vi "Needle_controller_tester.vi"() -> ()   [LabVIEW 2018]
uses:
  <vilib>/Analysis/baseanly.llb/A x Vector.vi
  <vilib>/Analysis/NI_AALBase.lvlib
panel:
  in  "Rate":u8(ring)=15 items=["ADC18_DATA_RATE_1_SPS", "ADC18_DATA_RATE_3_SPS", "ADC18_DATA_RATE_5_SPS", "ADC18_DATA_RATE_10_SPS", "ADC18_DATA_RATE_13_SPS", "ADC18_DATA_RATE_15_SPS", "ADC18_DATA_RATE_50_SPS", "ADC18_DATA_RATE_60_SPS", "ADC18_DATA_RATE_150_SPS", "ADC18_DATA_RATE_300_SPS", "ADC18_DATA_RATE_900_SPS", "ADC18_DATA_RATE_1800_SPS", "ADC18_DATA_RATE_2880_SPS", "ADC18_DATA_RATE_5760_SPS", "ADC18_DATA_RATE_11520_SPS", "ADC18_DATA_RATE_23040_SPS"]
  in  "Mode":u8(ring)=2 items=["CONTINUOUS", "CONTINUOUS 2", "SINGLE_CYCLE", "CONT_SINGLE_CYCLE"]
  in  "Set ADC Data Rate":bool
  in  "Samples To Average":u8=3
  in  "Get All Sensor Data Continuous":bool
  out "All Data 2":T1={"Time"=713, "FT Data"={"xForce"=0.14730099, "yForce"=0.008982421, "zForce"=0.2579272, "xTorque"=-0.9978087, "yTorque"=-0.58180696, "zTorque"=-0.619802}, "Encoder Data"={"xPos"=0.0, "yPos"=0.0, "zPos"=0.0}}
  out "Encoder Data":cluster{"xPos":sgl, "yPos":sgl, "zPos":sgl}
  in  "Get Encoder Sensor Data":bool
  out "All Data":T1={"Time"=992, "FT Data"={"xForce"=0.14789405, "yForce"=0.009089709, "zForce"=0.2569944, "xTorque"=-0.9979577, "yTorque"=-0.58224803, "zTorque"=-0.6196828}, "Encoder Data"={"xPos"=0.0, "yPos"=0.0, "zPos"=0.0}}
  in  "Get All Sensor Data":bool
  in  "Set ADC Conversion Mode":bool
  in  "Check ADC":bool
  in  "Reset ADC":bool
  out "Calibrated":dbl[](array[numeric]) format="%.2f"
  out "Sensor Data":T2
  out "System Status":cluster{"boardState":u8}
  in  "Get FT Sensor Data":bool
  out "Error Code":T3(ring)
  out "Return FID":u8=4
  out "FID":u8=5
  in  "IP Address":string="192.168.5.101"
  out "System Info":T4={"fwVersion"="1.0", "pumpId"="NeedleController01", "ipAddr"="192.168.5.101", "macAddr"="3e:43:d3:26:35:fe"}
  out "error out":errorcluster
  in  "Get System Info":bool
  in  "Get System Status":bool
  in  "Stop":bool
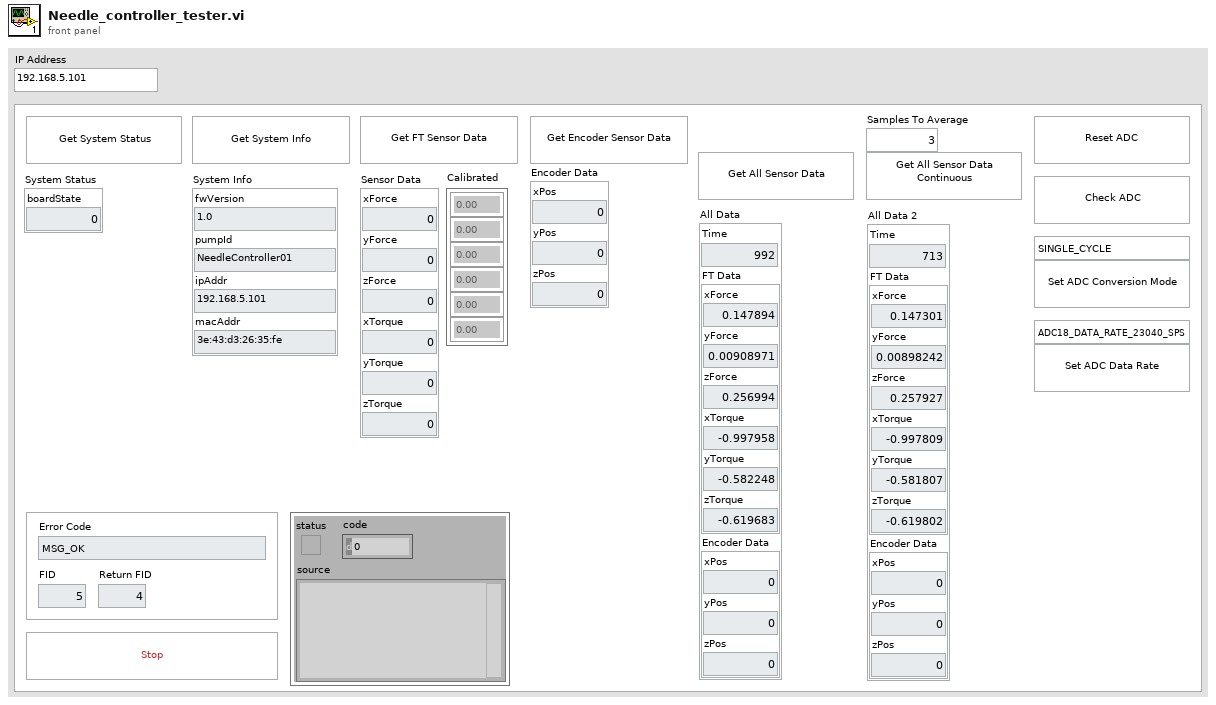
[diagram p1: front panel]
types:
  T1 = cluster{"Time":i32, "FT Data":cluster{"xForce":sgl, "yForce":sgl, "zForce":sgl, "xTorque":sgl, "yTorque":sgl, "zTorque":sgl}, "Encoder Data":cluster{"xPos":sgl, "yPos":sgl, "zPos":sgl}}
  T2 = cluster{"xForce":sgl, "yForce":sgl, "zForce":sgl, "xTorque":sgl, "yTorque":sgl, "zTorque":sgl}
  T3 = enum8{"MSG_OK", "MSG_ERROR_NOT_SUPPORTED", "MSG_ERROR_SENSOR_DISCONNECTED", "MSG_ERROR_READING_PENDING"}
  T4 = cluster{"fwVersion":string, "pumpId":string, "ipAddr":string, "macAddr":string}
  T5 = cluster{"fwVersion":string, "pumpId":string, "macAddr":string, "ipAddr":string}
  T6 = enum16{"big-endian, network order", "native, host order", "little-endian"}
  T7 = cluster{i32, "Sensor Data":cluster{"xForce":sgl, "yForce":sgl, "zForce":sgl, "xTorque":sgl, "yTorque":sgl, "zTorque":sgl}, "Sensor Data 2":cluster{"xForce":sgl, "yForce":sgl, "zForce":sgl}}
  T8 = cluster{"pumpState":i32, "suppliedVolume_ml":sgl, "flowRate_mlmin":sgl, "home":i32, "port":i32}
  T9 = cluster{"connection ID":refnum<k5>, "header length":u16}
  T10 = cluster{"boardState":u8, "tempSetpoint":sgl, "pH connected":bool, "Temp connected":bool, "pidOutput":dbl, "pidIntegral":dbl, "pidSetpoint":sgl, "pidStep":sgl, "pidMethod":u8}
  T11 = cluster{"header":cluster{"length":u16, "fid":u8, "error":u8}}
  T12 = cluster{"header":cluster{"length":u16, "fid":u8, "error":u8}, "Samples To Average":u8}
  T13 = cluster{"header":cluster{"length":u16, "fid":u8, "error":u8}, "Mode":u8}
  T14 = cluster{"header":cluster{"length":u16, "fid":u8, "error":u8}, "Rate":u8}
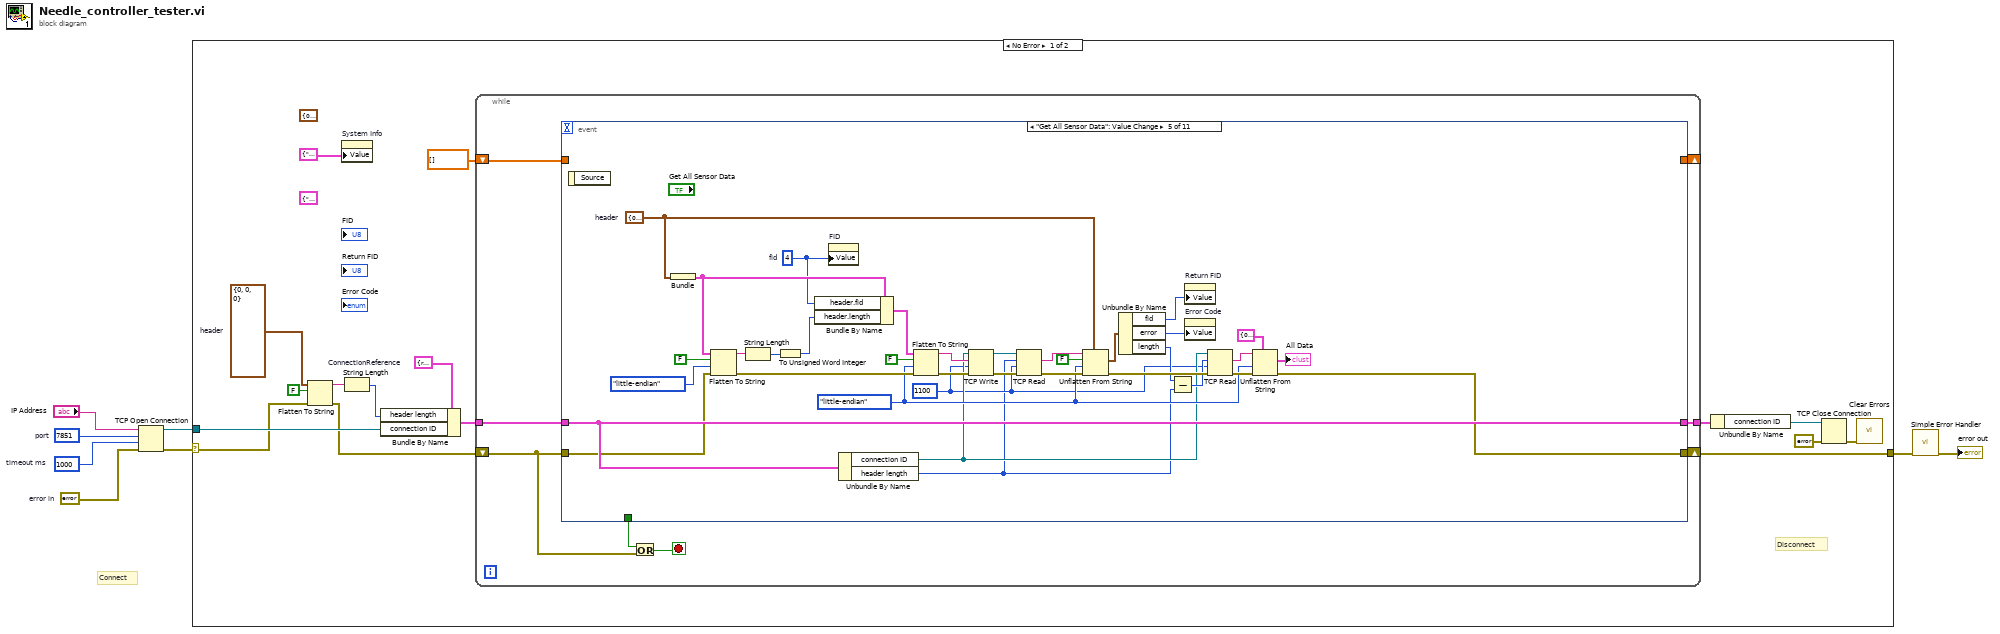
[diagram p0: block diagram]
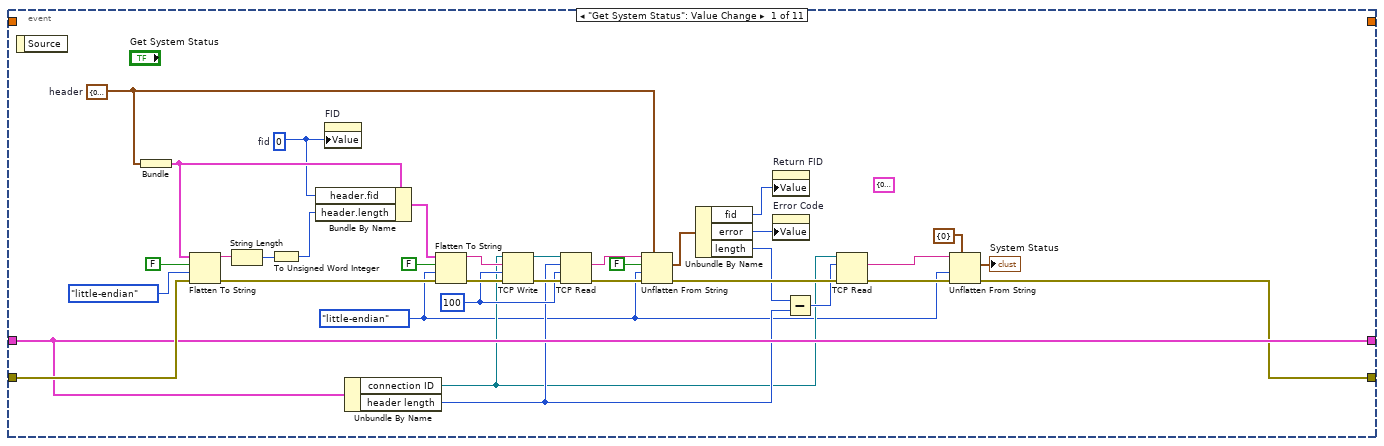
[diagram p2: hidden frame]
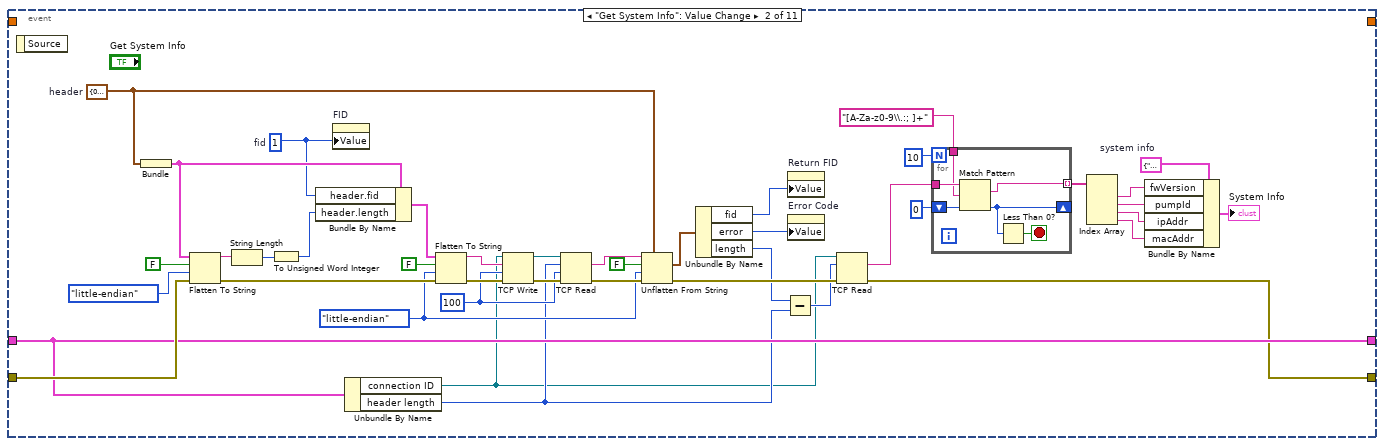
[diagram p3: hidden frame]
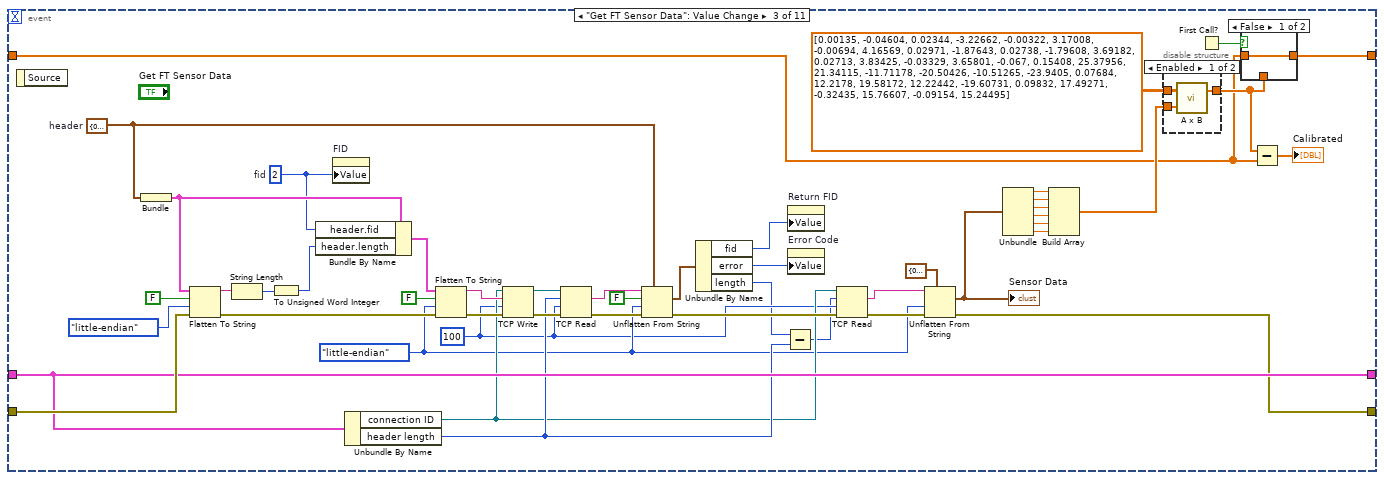
[diagram p4: hidden frame]
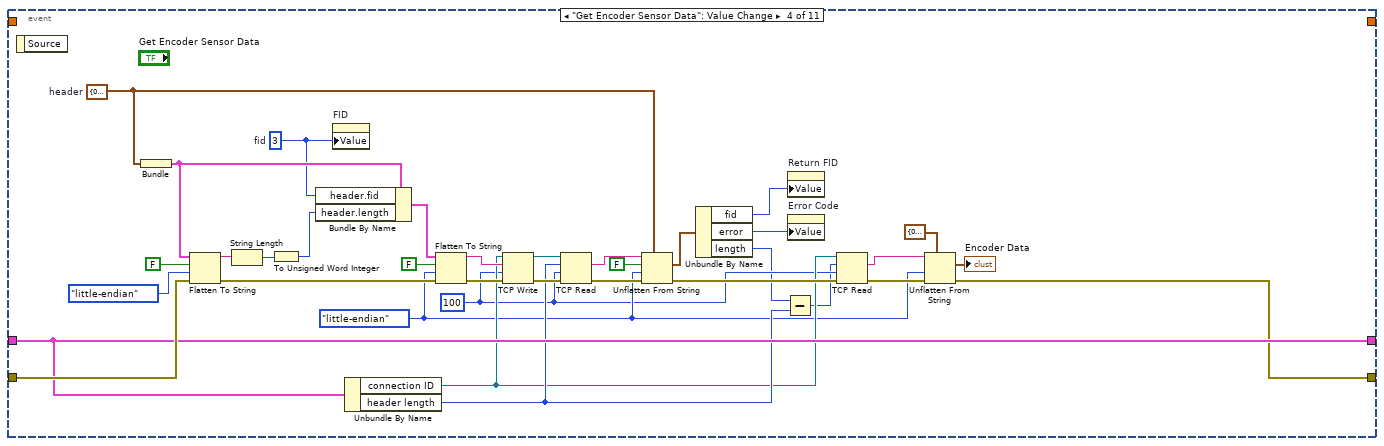
[diagram p7: hidden frame]
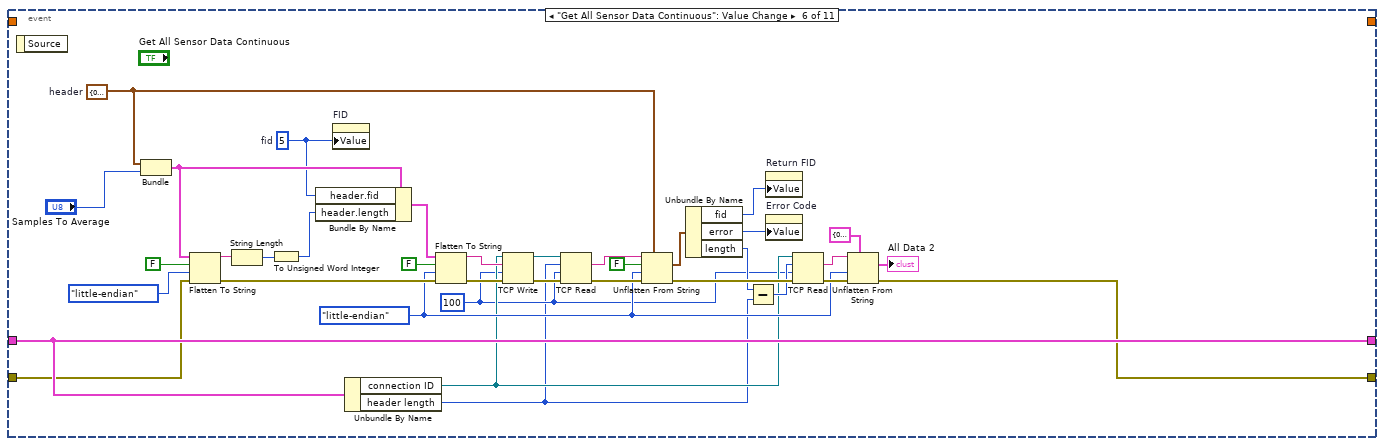
[diagram p8: hidden frame]
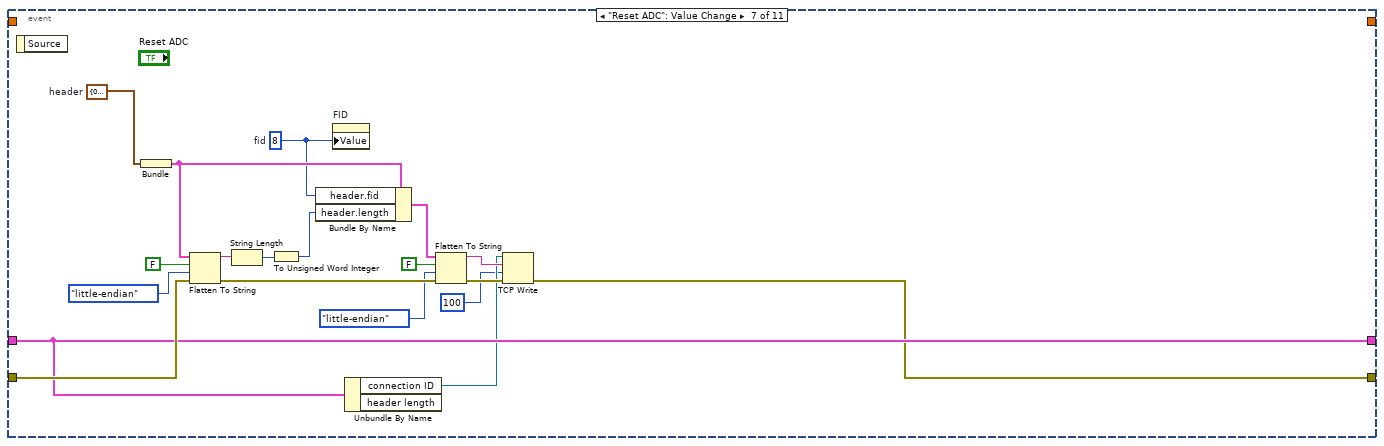
[diagram p9: hidden frame]
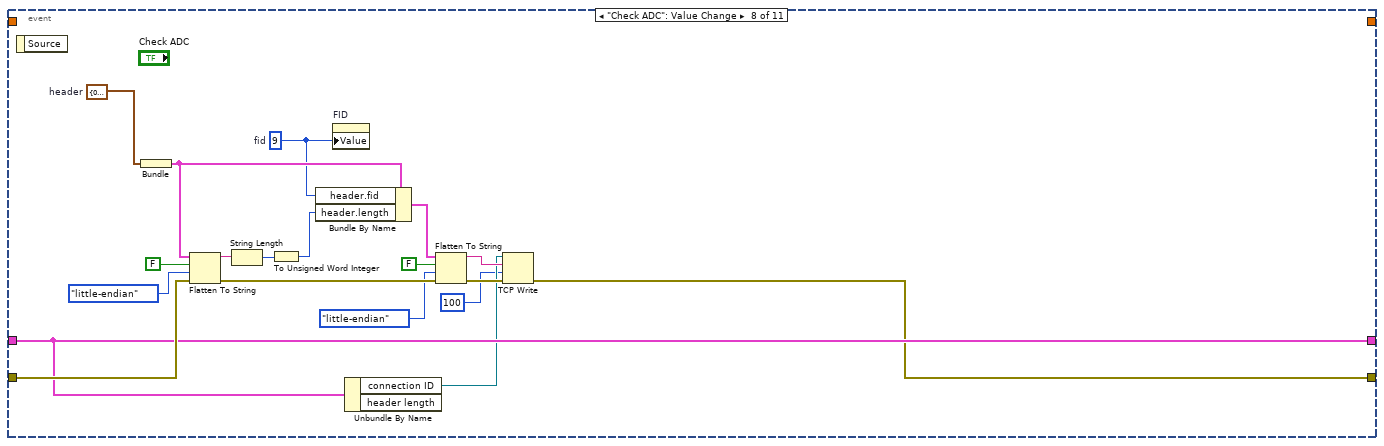
[diagram p10: hidden frame]
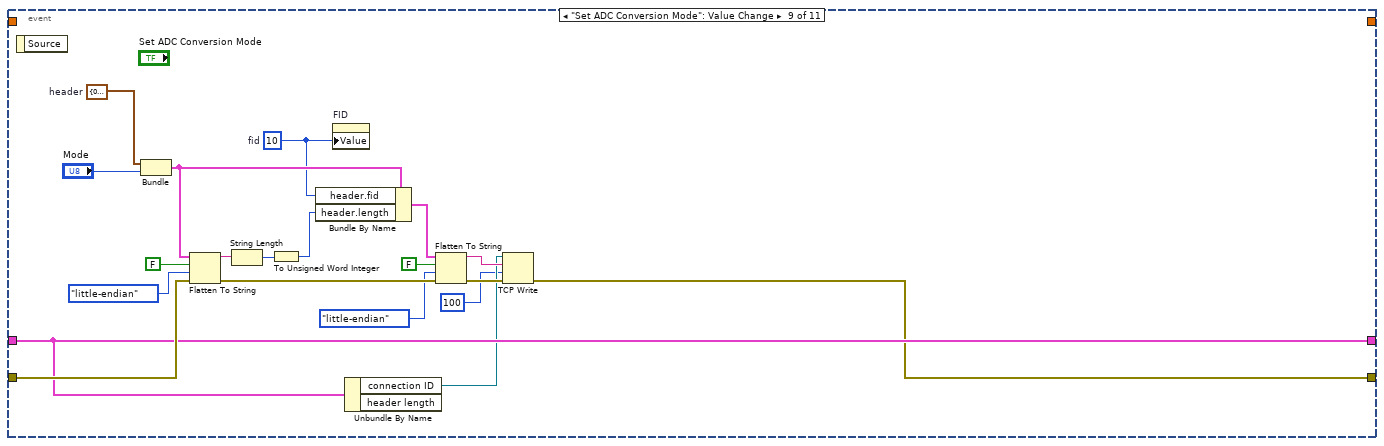
[diagram p11: hidden frame]
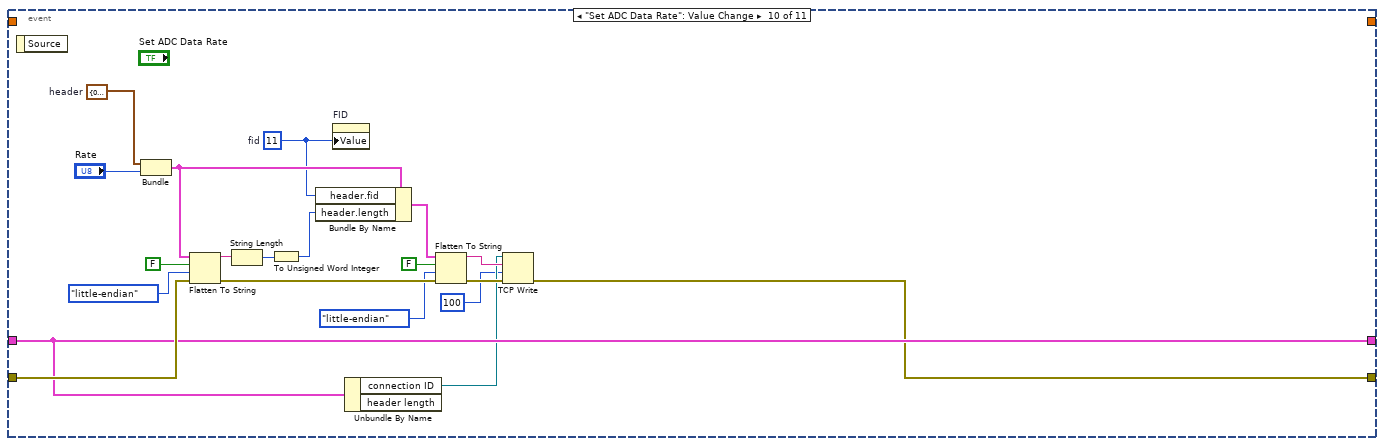
[diagram p12: hidden frame]
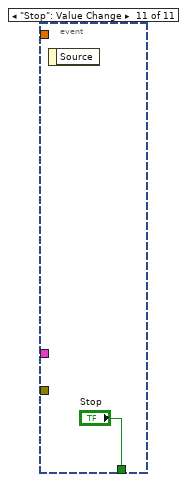
[diagram p13: hidden frame]
diagram:
  w6 = errorcluster {"status"=FALSE, "code"=0, "source"=""}  # error in
  w7 = 1000  # timeout ms
  w8 = u16 7851  # port
  # "Connect"
  n1 = TCP Open Connection(address="IP Address", remote port or service name=w8, timeout ms (60000)=w7, error in (no error)=w6) -> (connection ID=w5:refnum<k5>, error out=w1:errorcluster)  [unwired: 1 in]
  n2 = case shown="No Error" w1 {
    selector: w1 -> [w11 w355]
    tunnel: w5 -> [w20 _]
    tunnel: [w12 w355] -> w2
    frame No Error {
      (unwired) cluster{"axis":string, "stepPeriod (ms)":string} {"axis"="", "stepPeriod (ms)"=""} ("Return Motor Config")
      (unwired) T8 {"pumpState"=0, "suppliedVolume_ml"=0.0, "flowRate_mlmin"=0.0, "home"=0, "port"=0} ("Status")
      w19 = cluster{"length":u16, "fid":u8, "error":u8} {"length"=0, "fid"=0, "error"=0}  # header
      w21 = T9 {"connection ID"=refnum, "header length"=0}  # ConnectionReference
      # "Disconnect"
      n3 = Flatten To String(anything=w19, prepend array or string size? (T)=FALSE, error in (no error)=w11) -> (data string=w17:string, error out=w13:errorcluster)  [unwired: 1 in, 1 out]
      n4 = property on="System Info" class="Clust (strict)"("Value"=T5 {"fwVersion"="", "pumpId"="", "macAddr"="", "ipAddr"=""} ("system info")) -> ()  [unwired: 2 in, 2 out]
      n5 = String Length(string=w17) -> (length=w16:i32)
      n6 = Bundle By Name(cluster=w21, "header length"=w16, "connection ID"=w20) -> (w15:T9)
      n7 = while {
        tunnel: w15 -> [w32]
        tunnel: [w31] -> w14
        shift-right: [w30] -> w12
        shift-left: w13 -> [w28]
        shift-right: [w26] -> _
        shift-left: dbl[] [] ("A x Vector") -> [w25]
        stop <- w29 stop-if-true
        n8 = event shown="[4] \"Get All Sensor Data\": Value Change" {
          selector: _ -> [_ _ _ _ _ _ _ _ _ _ _]
          dyn-events: _ -> [_ _ _ _ _ _ _ _ _ _ _]
          timeout: _ -> [_ _ _ _ _ _ _ _ _ _ _]
          tunnel: w32 -> [w56 w98 w152 w193 w229 w265 w283 w302 w322 w342 _]
          tunnel: [w56 w98 w152 w193 w229 w265 w283 w302 w322 w342 _] -> w31
          tunnel: w28 -> [w57 w99 w153 w194 w206 w242 w284 w303 w323 w343 _]
          tunnel: [w39 w75 w136 w177 w207 w243 w276 w295 w315 w335 _] -> w30
          tunnel: [_ _ _ _ _ _ _ _ _ _ "Stop"] -> w27
          tunnel: [_ _ w119 _ _ _ _ _ _ _ _] -> w26
          tunnel: w25 -> [_ _ w117 _ _ _ _ _ _ _ _]
          event "Get System Status": Value Change {
            (unwired) T10 {"boardState"=0, "tempSetpoint"=0.0, "pH connected"=FALSE, "Temp connected"=FALSE, "pidOutput"=0.0, "pidIntegral"=0.0, "pidSetpoint"=0.0, "pidStep"=0.0, "pidMethod"=0} ("Status")
            w48 = cluster{"length":u16, "fid":u8, "error":u8} {"length"=0, "fid"=0, "error"=0}  # header
            w50 = 100 ("timeout ms (25000)")
            w36 = u8 0  # fid
            w38 = T6."little-endian" ("byte order (0:big-endian, network order)")
            n9 = event-data() -> ()  [unwired: 1 in, 1 out]
            n10 = Bundle("header"=w48) -> (w63:T11)  [unwired: 1 in]
            n11 = Flatten To String(anything=w63, prepend array or string size? (T)=FALSE, byte order (0:big-endian, network order)=T6."little-endian", error in (no error)=w57) -> (data string=w61:string, error out=w62:errorcluster)  [unwired: 1 out]
            n12 = String Length(string=w61) -> (length=w60:i32)
            n13 = To Unsigned Word Integer(number=w60) -> (unsigned 16bit integer=w59:u16)
            n14 = Bundle By Name(cluster=w63, "header.fid"=w36, "header.length"=w59) -> (w64:T11)
            n15 = property on="FID" class="DigNum (strict)"("Value"=w36) -> ()  [unwired: 2 in, 2 out]
            n16 = Unbundle By Name(w56) -> ("connection ID"=w42:refnum<k5>, "header length"=w44:u16)
            n17 = Flatten To String(anything=w64, prepend array or string size? (T)=FALSE, byte order (0:big-endian, network order)=w38, error in (no error)=w62) -> (data string=w66:string, error out=w67:errorcluster)  [unwired: 1 out]
            n18 = TCP Write(connection ID=w42, data in=w66, error in (no error)=w67, 9:w50) -> (connection ID out=w51:refnum<k5>, error out=w52:errorcluster)  [unwired: 1 out]
            n19 = TCP Read(connection ID=w51, bytes to read=w44, error in (no error)=w52, 9:w50) -> (data out=w53:string, error out=w54:errorcluster)  [unwired: 1 in, 1 out]
            n20 = Unflatten From String(type=w48, binary string=w53, data includes array or string size? (T)=FALSE, byte order (0:big-endian, network order)=w38, error in (no error)=w54) -> (value=w49:cluster{"length":u16, "fid":u8, "error":u8}, error out=w46:errorcluster)  [unwired: 1 out]
            n21 = Unbundle By Name(w49) -> ("fid"=w37:u8, "error"=w35:u8, "length"=w45:u16)
            n22 = property on="Return FID" class="DigNum (strict)"("Value"=w37) -> ()  [unwired: 2 in, 2 out]
            n23 = property on="Error Code" class="Enum (strict)"("Value"=w35) -> ()  [unwired: 2 in, 2 out]
            n24 = Subtract(x=w45, y=w44) -> (x-y=w43:u16)
            n25 = TCP Read(connection ID=w42, bytes to read=w43, error in (no error)=w46) -> (data out=w41:string, error out=w40:errorcluster)  [unwired: 2 in, 1 out]
            n26 = Unflatten From String(type=cluster{"boardState":u8} {"boardState"=0} ("System Status"), binary string=w41, byte order (0:big-endian, network order)=w38, error in (no error)=w40) -> (value=→"System Status":cluster{"boardState":u8}, error out=w39:errorcluster)  [unwired: 1 in, 1 out]
          }
          event "Get System Info": Value Change {
            w87 = T4 {"fwVersion"="", "pumpId"="", "ipAddr"="", "macAddr"=""}  # system info
            w89 = cluster{"length":u16, "fid":u8, "error":u8} {"length"=0, "fid"=0, "error"=0}  # header
            w92 = 100 ("timeout ms (25000)")
            w70 = u8 1  # fid
            w91 = T6."little-endian" ("byte order (0:big-endian, network order)")
            n27 = event-data() -> ()  [unwired: 1 in, 1 out]
            n28 = Bundle("header"=w89) -> (w105:T11)  [unwired: 1 in]
            n29 = Flatten To String(anything=w105, prepend array or string size? (T)=FALSE, byte order (0:big-endian, network order)=T6."little-endian", error in (no error)=w99) -> (data string=w103:string, error out=w104:errorcluster)  [unwired: 1 out]
            n30 = String Length(string=w103) -> (length=w102:i32)
            n31 = To Unsigned Word Integer(number=w102) -> (unsigned 16bit integer=w101:u16)
            n32 = Bundle By Name(cluster=w105, "header.fid"=w70, "header.length"=w101) -> (w106:T11)
            n33 = property on="FID" class="DigNum (strict)"("Value"=w70) -> ()  [unwired: 2 in, 2 out]
            n34 = Unbundle By Name(w98) -> ("connection ID"=w71:refnum<k5>, "header length"=w73:u16)
            n35 = Flatten To String(anything=w106, prepend array or string size? (T)=FALSE, byte order (0:big-endian, network order)=w91, error in (no error)=w104) -> (data string=w108:string, error out=w109:errorcluster)  [unwired: 1 out]
            n36 = TCP Write(connection ID=w71, data in=w108, error in (no error)=w109, 9:w92) -> (connection ID out=w93:refnum<k5>, error out=w94:errorcluster)  [unwired: 1 out]
            n37 = TCP Read(connection ID=w93, bytes to read=w73, error in (no error)=w94, 9:w92) -> (data out=w95:string, error out=w96:errorcluster)  [unwired: 1 in, 1 out]
            n38 = Unflatten From String(type=w89, binary string=w95, data includes array or string size? (T)=FALSE, byte order (0:big-endian, network order)=w91, error in (no error)=w96) -> (value=w90:cluster{"length":u16, "fid":u8, "error":u8}, error out=w77:errorcluster)  [unwired: 1 out]
            n39 = Unbundle By Name(w90) -> ("fid"=w69:u8, "error"=w68:u8, "length"=w74:u16)
            n40 = Subtract(x=w74, y=w73) -> (x-y=w72:u16)
            n41 = property on="Return FID" class="DigNum (strict)"("Value"=w69) -> ()  [unwired: 2 in, 2 out]
            n42 = property on="Error Code" class="Enum (strict)"("Value"=w68) -> ()  [unwired: 2 in, 2 out]
            n43 = TCP Read(connection ID=w71, bytes to read=w72, error in (no error)=w77) -> (data out=w85:string, error out=w75:errorcluster)  [unwired: 2 in, 1 out]
            n44 = for {
              N: 10 -> [_]
              shift-right: [w111] -> _
              shift-left: 0 ("offset past match") -> [w115]
              tunnel: w85 -> [w114]
              tunnel: "[A-Za-z0-9\\.:; ]+" ("regular expression") -> [w113]
              tunnel: [w110] -> w82 mode=indexing
              stop <- w112 stop-if-true
              n45 = Match Pattern(string=w114, regular expression=w113, offset (0)=w115) -> (match substring=w110:string, offset past match=w111:i32)  [unwired: 2 out]
              n46 = Less Than 0?(x=w111) -> (x < 0?=w112:bool)
            }
            n47 = Index Array(array=w82) -> (element #1=w81:string, element #2=w80:string, element #3=w79:string, element #4=w78:string)  [unwired: 4 in]
            n48 = Bundle By Name(cluster=w87, "fwVersion"=w81, "pumpId"=w80, "ipAddr"=w79, "macAddr"=w78) -> (→"System Info":T4)
          }
          event "Get FT Sensor Data": Value Change {
            w145 = cluster{"length":u16, "fid":u8, "error":u8} {"length"=0, "fid"=0, "error"=0}  # header
            w133 = 100 ("timeout ms (25000)")
            w140 = u8 2  # fid
            w134 = T6."little-endian" ("byte order (0:big-endian, network order)")
            n49 = event-data() -> ()  [unwired: 1 in, 1 out]
            n50 = Bundle("header"=w145) -> (w159:T11)  [unwired: 1 in]
            n51 = Flatten To String(anything=w159, prepend array or string size? (T)=FALSE, byte order (0:big-endian, network order)=T6."little-endian", error in (no error)=w153) -> (data string=w157:string, error out=w158:errorcluster)  [unwired: 1 out]
            n52 = String Length(string=w157) -> (length=w156:i32)
            n53 = To Unsigned Word Integer(number=w156) -> (unsigned 16bit integer=w155:u16)
            n54 = Bundle By Name(cluster=w159, "header.fid"=w140, "header.length"=w155) -> (w160:T11)
            n55 = property on="FID" class="DigNum (strict)"("Value"=w140) -> ()  [unwired: 2 in, 2 out]
            n56 = Unbundle By Name(w152) -> ("connection ID"=w141:refnum<k5>, "header length"=w142:u16)
            n57 = Flatten To String(anything=w160, prepend array or string size? (T)=FALSE, byte order (0:big-endian, network order)=w134, error in (no error)=w158) -> (data string=w162:string, error out=w163:errorcluster)  [unwired: 1 out]
            n58 = TCP Write(connection ID=w141, data in=w162, error in (no error)=w163, 9:w133) -> (connection ID out=w147:refnum<k5>, error out=w148:errorcluster)  [unwired: 1 out]
            n59 = TCP Read(connection ID=w147, bytes to read=w142, error in (no error)=w148, 9:w133) -> (data out=w149:string, error out=w150:errorcluster)  [unwired: 1 in, 1 out]
            n60 = Unflatten From String(type=w145, binary string=w149, data includes array or string size? (T)=FALSE, byte order (0:big-endian, network order)=w134, error in (no error)=w150) -> (value=w146:cluster{"length":u16, "fid":u8, "error":u8}, error out=w143:errorcluster)  [unwired: 1 out]
            n61 = Unbundle By Name(w146) -> ("fid"=w139:u8, "error"=w138:u8, "length"=w130:u16)
            n62 = Subtract(x=w130, y=w142) -> (x-y=w131:u16)
            n63 = property on="Return FID" class="DigNum (strict)"("Value"=w139) -> ()  [unwired: 2 in, 2 out]
            n64 = property on="Error Code" class="Enum (strict)"("Value"=w138) -> ()  [unwired: 2 in, 2 out]
            n65 = TCP Read(connection ID=w141, bytes to read=w131, error in (no error)=w143, 9:w133) -> (data out=w135:string, error out=w137:errorcluster)  [unwired: 1 in, 1 out]
            n66 = Unflatten From String(type=T2 {"xForce"=0.0, "yForce"=0.0, "zForce"=0.0, "xTorque"=0.0, "yTorque"=0.0, "zTorque"=0.0} ("Sensor Data"), binary string=w135, byte order (0:big-endian, network order)=w134, error in (no error)=w137) -> (value=w128:T2, error out=w136:errorcluster)  [unwired: 1 in, 1 out]
            "Sensor Data" <- w128
            n67 = Unbundle(w128) -> ("xForce"=w127:sgl, "yForce"=w122:sgl, "zForce"=w123:sgl, "xTorque"=w124:sgl, "yTorque"=w125:sgl, "zTorque"=w126:sgl)
            n68 = Build Array(w127, w122, w123, w124, w125, w126) -> (w121:sgl[])
            n69 = disable-structure shown="Enabled" {
              disable-tunnel: dbl[][] [[0.00135, -0.04604, 0.02344, -3.22662, -0.00322, 3.17008], [-0.00694, 4.16569, 0.02971, -1.87643, 0.02738, -1.79608], [3.69182, 0.02713, 3.83425, -0.03329, 3.65801, -0.067], [0.15408, 25.37956, 21.34115, -11.71178, -20.50426, -10.51265], [-23.9405, 0.07684, 12.2178, 19.58172, 12.22442, -19.60731], [0.09832, 17.49271, -0.32435, 15.76607, -0.09154, 15.24495]] ("Calibration Matrix") -> [w166 _]
              disable-tunnel: w121 -> [w165 w167]
              disable-tunnel: [w164 w167] -> w118
              frame Enabled {
                n70 = call-poly <vilib>:"A x B.vi"("Vector"=w165, "A"=w166) -> ("A x Vector"=w164:dbl[])  [unwired: 1 out]
              }
              frame Disabled {
              }
            }
            n71 = First Call?() -> (First Call?: T/F=w116:bool)
            n72 = case shown="False" w116 {
              tunnel: [w168 w169] -> w119
              tunnel: w118 -> [_ w169]
              tunnel: w117 -> [w168 _]
              frame False {
              }
              frame True {
              }
            }
            n73 = Subtract(x=w118, y=w117) -> (x-y=→"Calibrated":dbl[])
          }
          event "Get Encoder Sensor Data": Value Change {
            w186 = cluster{"length":u16, "fid":u8, "error":u8} {"length"=0, "fid"=0, "error"=0}  # header
            w174 = 100 ("timeout ms (25000)")
            w181 = u8 3  # fid
            w175 = T6."little-endian" ("byte order (0:big-endian, network order)")
            n74 = event-data() -> ()  [unwired: 1 in, 1 out]
            n75 = Bundle("header"=w186) -> (w200:T11)  [unwired: 1 in]
            n76 = Flatten To String(anything=w200, prepend array or string size? (T)=FALSE, byte order (0:big-endian, network order)=T6."little-endian", error in (no error)=w194) -> (data string=w198:string, error out=w199:errorcluster)  [unwired: 1 out]
            n77 = String Length(string=w198) -> (length=w197:i32)
            n78 = To Unsigned Word Integer(number=w197) -> (unsigned 16bit integer=w196:u16)
            n79 = Bundle By Name(cluster=w200, "header.fid"=w181, "header.length"=w196) -> (w201:T11)
            n80 = property on="FID" class="DigNum (strict)"("Value"=w181) -> ()  [unwired: 2 in, 2 out]
            n81 = Unbundle By Name(w193) -> ("connection ID"=w182:refnum<k5>, "header length"=w183:u16)
            n82 = Flatten To String(anything=w201, prepend array or string size? (T)=FALSE, byte order (0:big-endian, network order)=w175, error in (no error)=w199) -> (data string=w203:string, error out=w204:errorcluster)  [unwired: 1 out]
            n83 = TCP Write(connection ID=w182, data in=w203, error in (no error)=w204, 9:w174) -> (connection ID out=w188:refnum<k5>, error out=w189:errorcluster)  [unwired: 1 out]
            n84 = TCP Read(connection ID=w188, bytes to read=w183, error in (no error)=w189, 9:w174) -> (data out=w190:string, error out=w191:errorcluster)  [unwired: 1 in, 1 out]
            n85 = Unflatten From String(type=w186, binary string=w190, data includes array or string size? (T)=FALSE, byte order (0:big-endian, network order)=w175, error in (no error)=w191) -> (value=w187:cluster{"length":u16, "fid":u8, "error":u8}, error out=w184:errorcluster)  [unwired: 1 out]
            n86 = Unbundle By Name(w187) -> ("fid"=w180:u8, "error"=w179:u8, "length"=w171:u16)
            n87 = Subtract(x=w171, y=w183) -> (x-y=w172:u16)
            n88 = property on="Return FID" class="DigNum (strict)"("Value"=w180) -> ()  [unwired: 2 in, 2 out]
            n89 = property on="Error Code" class="Enum (strict)"("Value"=w179) -> ()  [unwired: 2 in, 2 out]
            n90 = TCP Read(connection ID=w182, bytes to read=w172, error in (no error)=w184, 9:w174) -> (data out=w176:string, error out=w178:errorcluster)  [unwired: 1 in, 1 out]
            n91 = Unflatten From String(type=cluster{"xPos":sgl, "yPos":sgl, "zPos":sgl} {"xPos"=0.0, "yPos"=0.0, "zPos"=0.0} ("Sensor Data"), binary string=w176, byte order (0:big-endian, network order)=w175, error in (no error)=w178) -> (value=→"Encoder Data":cluster{"xPos":sgl, "yPos":sgl, "zPos":sgl}, error out=w177:errorcluster)  [unwired: 1 in, 1 out]
          }
          event "Get All Sensor Data": Value Change {
            w213 = cluster{"length":u16, "fid":u8, "error":u8} {"length"=0, "fid"=0, "error"=0}  # header
            w210 = 1100 ("timeout ms (25000)")
            w220 = u8 4  # fid
            w212 = T6."little-endian" ("byte order (0:big-endian, network order)")
            n92 = event-data() -> ()  [unwired: 1 in, 1 out]
            n93 = Bundle("header"=w213) -> (w235:T11)  [unwired: 1 in]
            n94 = Flatten To String(anything=w235, prepend array or string size? (T)=FALSE, byte order (0:big-endian, network order)=T6."little-endian", error in (no error)=w206) -> (data string=w233:string, error out=w234:errorcluster)  [unwired: 1 out]
            n95 = String Length(string=w233) -> (length=w232:i32)
            n96 = To Unsigned Word Integer(number=w232) -> (unsigned 16bit integer=w231:u16)
            n97 = Bundle By Name(cluster=w235, "header.fid"=w220, "header.length"=w231) -> (w236:T11)
            n98 = property on="FID" class="DigNum (strict)"("Value"=w220) -> ()  [unwired: 2 in, 2 out]
            n99 = Unbundle By Name(w229) -> ("connection ID"=w211:refnum<k5>, "header length"=w209:u16)
            n100 = Flatten To String(anything=w236, prepend array or string size? (T)=FALSE, byte order (0:big-endian, network order)=w212, error in (no error)=w234) -> (data string=w238:string, error out=w239:errorcluster)  [unwired: 1 out]
            n101 = TCP Write(connection ID=w211, data in=w238, error in (no error)=w239, 9:w210) -> (connection ID out=w224:refnum<k5>, error out=w225:errorcluster)  [unwired: 1 out]
            n102 = TCP Read(connection ID=w224, bytes to read=w209, error in (no error)=w225, 9:w210) -> (data out=w226:string, error out=w227:errorcluster)  [unwired: 1 in, 1 out]
            n103 = Unflatten From String(type=w213, binary string=w226, data includes array or string size? (T)=FALSE, byte order (0:big-endian, network order)=w212, error in (no error)=w227) -> (value=w223:cluster{"length":u16, "fid":u8, "error":u8}, error out=w221:errorcluster)  [unwired: 1 out]
            n104 = Unbundle By Name(w223) -> ("fid"=w219:u8, "error"=w218:u8, "length"=w214:u16)
            n105 = Subtract(x=w214, y=w209) -> (x-y=w215:u16)
            n106 = property on="Return FID" class="DigNum (strict)"("Value"=w219) -> ()  [unwired: 2 in, 2 out]
            n107 = property on="Error Code" class="Enum (strict)"("Value"=w218) -> ()  [unwired: 2 in, 2 out]
            n108 = TCP Read(connection ID=w211, bytes to read=w215, error in (no error)=w221, 9:w210) -> (data out=w216:string, error out=w217:errorcluster)  [unwired: 1 in, 1 out]
            n109 = Unflatten From String(type=T7 {0, "Sensor Data"={"xForce"=0.0, "yForce"=0.0, "zForce"=0.0, "xTorque"=0.0, "yTorque"=0.0, "zTorque"=0.0}, "Sensor Data 2"={"xForce"=0.0, "yForce"=0.0, "zForce"=0.0}}, binary string=w216, byte order (0:big-endian, network order)=w212, error in (no error)=w217) -> (value=→"All Data":T7, error out=w207:errorcluster)  [unwired: 1 in, 1 out]
          }
          event "Get All Sensor Data Continuous": Value Change {
            w249 = cluster{"length":u16, "fid":u8, "error":u8} {"length"=0, "fid"=0, "error"=0}  # header
            w246 = 100 ("timeout ms (25000)")
            w256 = u8 5  # fid
            w248 = T6."little-endian" ("byte order (0:big-endian, network order)")
            n110 = event-data() -> ()  [unwired: 1 in, 1 out]
            n111 = Bundle("header"=w249, "Samples To Average"="Samples To Average") -> (w271:T12)  [unwired: 1 in]
            n112 = Flatten To String(anything=w271, prepend array or string size? (T)=FALSE, byte order (0:big-endian, network order)=T6."little-endian", error in (no error)=w242) -> (data string=w269:string, error out=w270:errorcluster)  [unwired: 1 out]
            n113 = String Length(string=w269) -> (length=w268:i32)
            n114 = To Unsigned Word Integer(number=w268) -> (unsigned 16bit integer=w267:u16)
            n115 = Bundle By Name(cluster=w271, "header.fid"=w256, "header.length"=w267) -> (w272:T12)
            n116 = property on="FID" class="DigNum (strict)"("Value"=w256) -> ()  [unwired: 2 in, 2 out]
            n117 = Unbundle By Name(w265) -> ("connection ID"=w247:refnum<k5>, "header length"=w245:u16)
            n118 = Flatten To String(anything=w272, prepend array or string size? (T)=FALSE, byte order (0:big-endian, network order)=w248, error in (no error)=w270) -> (data string=w274:string, error out=w275:errorcluster)  [unwired: 1 out]
            n119 = TCP Write(connection ID=w247, data in=w274, error in (no error)=w275, 9:w246) -> (connection ID out=w260:refnum<k5>, error out=w261:errorcluster)  [unwired: 1 out]
            n120 = TCP Read(connection ID=w260, bytes to read=w245, error in (no error)=w261, 9:w246) -> (data out=w262:string, error out=w263:errorcluster)  [unwired: 1 in, 1 out]
            n121 = Unflatten From String(type=w249, binary string=w262, data includes array or string size? (T)=FALSE, byte order (0:big-endian, network order)=w248, error in (no error)=w263) -> (value=w259:cluster{"length":u16, "fid":u8, "error":u8}, error out=w257:errorcluster)  [unwired: 1 out]
            n122 = Unbundle By Name(w259) -> ("fid"=w255:u8, "error"=w254:u8, "length"=w250:u16)
            n123 = Subtract(x=w250, y=w245) -> (x-y=w251:u16)
            n124 = property on="Return FID" class="DigNum (strict)"("Value"=w255) -> ()  [unwired: 2 in, 2 out]
            n125 = property on="Error Code" class="Enum (strict)"("Value"=w254) -> ()  [unwired: 2 in, 2 out]
            n126 = TCP Read(connection ID=w247, bytes to read=w251, error in (no error)=w257, 9:w246) -> (data out=w252:string, error out=w253:errorcluster)  [unwired: 1 in, 1 out]
            n127 = Unflatten From String(type=T7 {0, "Sensor Data"={"xForce"=0.0, "yForce"=0.0, "zForce"=0.0, "xTorque"=0.0, "yTorque"=0.0, "zTorque"=0.0}, "Sensor Data 2"={"xForce"=0.0, "yForce"=0.0, "zForce"=0.0}}, binary string=w252, byte order (0:big-endian, network order)=w248, error in (no error)=w253) -> (value=→"All Data 2":T7, error out=w243:errorcluster)  [unwired: 1 in, 1 out]
          }
          event "Reset ADC": Value Change {
            w282 = cluster{"length":u16, "fid":u8, "error":u8} {"length"=0, "fid"=0, "error"=0}  # header
            w279 = u8 8  # fid
            n128 = event-data() -> ()  [unwired: 1 in, 1 out]
            n129 = Bundle("header"=w282) -> (w290:T11)  [unwired: 1 in]
            n130 = Flatten To String(anything=w290, prepend array or string size? (T)=FALSE, byte order (0:big-endian, network order)=T6."little-endian", error in (no error)=w284) -> (data string=w288:string, error out=w289:errorcluster)  [unwired: 1 out]
            n131 = String Length(string=w288) -> (length=w287:i32)
            n132 = To Unsigned Word Integer(number=w287) -> (unsigned 16bit integer=w286:u16)
            n133 = Bundle By Name(cluster=w290, "header.fid"=w279, "header.length"=w286) -> (w291:T11)
            n134 = property on="FID" class="DigNum (strict)"("Value"=w279) -> ()  [unwired: 2 in, 2 out]
            n135 = Unbundle By Name(w283) -> ("connection ID"=w280:refnum<k5>)  [unwired: 1 out]
            n136 = Flatten To String(anything=w291, prepend array or string size? (T)=FALSE, byte order (0:big-endian, network order)=T6."little-endian", error in (no error)=w289) -> (data string=w293:string, error out=w294:errorcluster)  [unwired: 1 out]
            n137 = TCP Write(connection ID=w280, data in=w293, error in (no error)=w294, 9:100 ("timeout ms (25000)")) -> (error out=w276:errorcluster)  [unwired: 2 out]
          }
          event "Check ADC": Value Change {
            w301 = cluster{"length":u16, "fid":u8, "error":u8} {"length"=0, "fid"=0, "error"=0}  # header
            w298 = u8 9  # fid
            n138 = event-data() -> ()  [unwired: 1 in, 1 out]
            n139 = Bundle("header"=w301) -> (w309:T11)  [unwired: 1 in]
            n140 = Flatten To String(anything=w309, prepend array or string size? (T)=FALSE, byte order (0:big-endian, network order)=T6."little-endian", error in (no error)=w303) -> (data string=w307:string, error out=w308:errorcluster)  [unwired: 1 out]
            n141 = String Length(string=w307) -> (length=w306:i32)
            n142 = To Unsigned Word Integer(number=w306) -> (unsigned 16bit integer=w305:u16)
            n143 = Bundle By Name(cluster=w309, "header.fid"=w298, "header.length"=w305) -> (w310:T11)
            n144 = property on="FID" class="DigNum (strict)"("Value"=w298) -> ()  [unwired: 2 in, 2 out]
            n145 = Unbundle By Name(w302) -> ("connection ID"=w299:refnum<k5>)  [unwired: 1 out]
            n146 = Flatten To String(anything=w310, prepend array or string size? (T)=FALSE, byte order (0:big-endian, network order)=T6."little-endian", error in (no error)=w308) -> (data string=w312:string, error out=w313:errorcluster)  [unwired: 1 out]
            n147 = TCP Write(connection ID=w299, data in=w312, error in (no error)=w313, 9:100 ("timeout ms (25000)")) -> (error out=w295:errorcluster)  [unwired: 2 out]
          }
          event "Set ADC Conversion Mode": Value Change {
            w321 = cluster{"length":u16, "fid":u8, "error":u8} {"length"=0, "fid"=0, "error"=0}  # header
            w318 = u8 10  # fid
            n148 = event-data() -> ()  [unwired: 1 in, 1 out]
            n149 = Bundle("header"=w321, "Mode"="Mode") -> (w329:T13)  [unwired: 1 in]
            n150 = Flatten To String(anything=w329, prepend array or string size? (T)=FALSE, byte order (0:big-endian, network order)=T6."little-endian", error in (no error)=w323) -> (data string=w327:string, error out=w328:errorcluster)  [unwired: 1 out]
            n151 = String Length(string=w327) -> (length=w326:i32)
            n152 = To Unsigned Word Integer(number=w326) -> (unsigned 16bit integer=w325:u16)
            n153 = Bundle By Name(cluster=w329, "header.fid"=w318, "header.length"=w325) -> (w330:T13)
            n154 = property on="FID" class="DigNum (strict)"("Value"=w318) -> ()  [unwired: 2 in, 2 out]
            n155 = Unbundle By Name(w322) -> ("connection ID"=w319:refnum<k5>)  [unwired: 1 out]
            n156 = Flatten To String(anything=w330, prepend array or string size? (T)=FALSE, byte order (0:big-endian, network order)=T6."little-endian", error in (no error)=w328) -> (data string=w332:string, error out=w333:errorcluster)  [unwired: 1 out]
            n157 = TCP Write(connection ID=w319, data in=w332, error in (no error)=w333, 9:100 ("timeout ms (25000)")) -> (error out=w315:errorcluster)  [unwired: 2 out]
          }
          event "Set ADC Data Rate": Value Change {
            w341 = cluster{"length":u16, "fid":u8, "error":u8} {"length"=0, "fid"=0, "error"=0}  # header
            w338 = u8 11  # fid
            n158 = event-data() -> ()  [unwired: 1 in, 1 out]
            n159 = Bundle("header"=w341, "Rate"="Rate") -> (w349:T14)  [unwired: 1 in]
            n160 = Flatten To String(anything=w349, prepend array or string size? (T)=FALSE, byte order (0:big-endian, network order)=T6."little-endian", error in (no error)=w343) -> (data string=w347:string, error out=w348:errorcluster)  [unwired: 1 out]
            n161 = String Length(string=w347) -> (length=w346:i32)
            n162 = To Unsigned Word Integer(number=w346) -> (unsigned 16bit integer=w345:u16)
            n163 = Bundle By Name(cluster=w349, "header.fid"=w338, "header.length"=w345) -> (w350:T14)
            n164 = property on="FID" class="DigNum (strict)"("Value"=w338) -> ()  [unwired: 2 in, 2 out]
            n165 = Unbundle By Name(w342) -> ("connection ID"=w339:refnum<k5>)  [unwired: 1 out]
            n166 = Flatten To String(anything=w350, prepend array or string size? (T)=FALSE, byte order (0:big-endian, network order)=T6."little-endian", error in (no error)=w348) -> (data string=w352:string, error out=w353:errorcluster)  [unwired: 1 out]
            n167 = TCP Write(connection ID=w339, data in=w352, error in (no error)=w353, 9:100 ("timeout ms (25000)")) -> (error out=w335:errorcluster)  [unwired: 2 out]
          }
          event "Stop": Value Change {
            n168 = event-data() -> ()  [unwired: 1 in, 1 out]
          }
        }
        n169 = Or(x=w27, y=w28) -> (x .or. y?=w29:bool)
      }
      n170 = Unbundle By Name(w14) -> ("connection ID"=w22:refnum<k5>)
      n171 = TCP Close Connection(connection ID=w22, error in (no error)=errorcluster {"status"=FALSE, "code"=0, "source"=""}) -> (error out=w23:errorcluster)  [unwired: 1 in, 1 out]
      n172 = call <vilib>:"Clear Errors.vi"("error in (no error)"=w23) -> ()  [unwired: 5 in, 2 out]
    }
    frame Error {
    }
  }
  n173 = call <vilib>:"Simple Error Handler.vi"("error in (no error)"=w2) -> ("error out"=→"error out":errorcluster)  [unwired: 4 in, 4 out]
